vi "input and personal tax calc .vi"(8 "error in (no error)":errorcluster, 11 "Tax_calculation in":refnum<class "Tax_calculation.lvclass">) -> (0 "error out":errorcluster, 3 "Tax_calculation out":refnum<class "Tax_calculation.lvclass">)   [LabVIEW 2016, in "Tax_calculation.lvclass"]
uses:
  Tax_calculation.lvclass
  Tax_calculation.lvclass/Tax_calculation.ctl
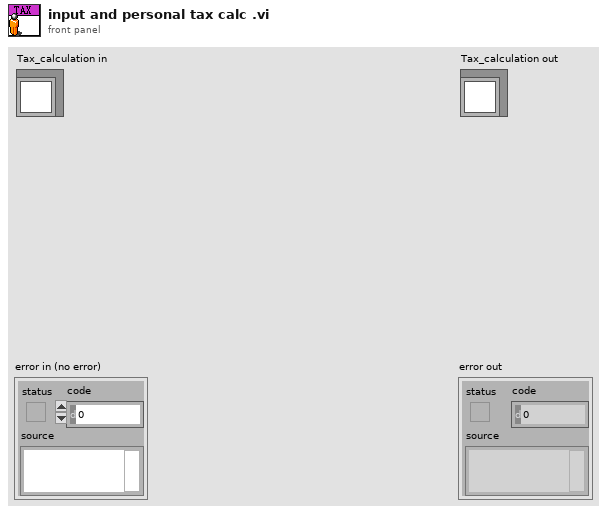
[diagram p1: front panel]
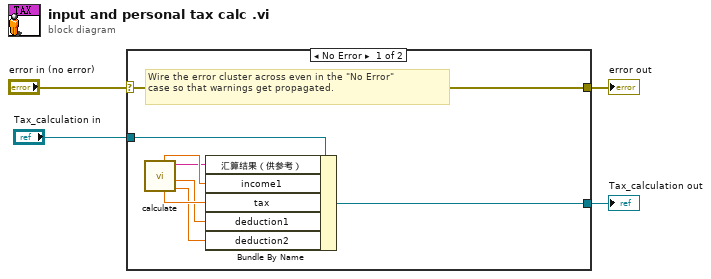
[diagram p0: block diagram]
diagram:
  n1 = case shown="No Error" "error in (no error)" {
    selector: "error in (no error)" -> [w12 w14]
    tunnel: [w12 w14] -> w3
    tunnel: [w5 w13] -> w1
    tunnel: "Tax_calculation in" -> [w7 w13]
    frame No Error {
      # "Wire the error cluster across even in the \"No Error\"\ncase so that warnings get propagated."
      n2 = call "calculate.vi"() -> ("抵扣2"=w8:dbl, "抵扣1"=w9:dbl, "汇算结果（供参考）"=w6:string, "税"=w11:dbl, "总收入"=w10:dbl)  [unwired: 7 in]
      n3 = Bundle By Name(cluster=w7, "汇算结果（供参考）"=w6, "income1"=w10, "tax"=w11, "deduction1"=w9, "deduction2"=w8) -> (w5:refnum<class "Tax_calculation.lvclass">)
    }
    frame Error {
    }
  }
  "error out" <- w3
  "Tax_calculation out" <- w1
